vi "CRIO_State2String.vi"(8 "error in (no error)":errorcluster, 11 "Curr State":T1) -> (0 "error out":errorcluster, 3 "State Str":string)   [LabVIEW 2017]
uses:
  CRIO_StateEnum.ctl
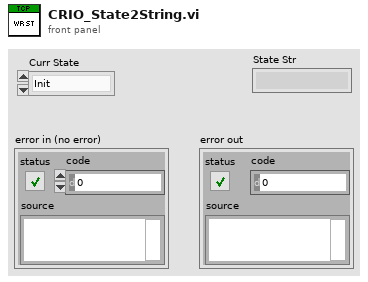
[diagram p1: front panel]
types:
  T1 = typedef "CRIO_StateEnum.ctl" = enum16{"Init", "Listen", "Wait", "Setup", "Ready to Launch", "Start Flight", "Accelerating", "Coasting", "Braking", "End Flight", "Loading", "Stop"}
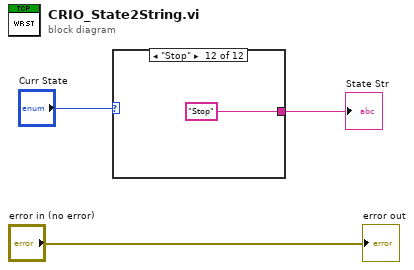
[diagram p0: block diagram]
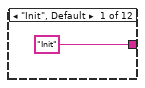
[diagram p2: hidden frame]
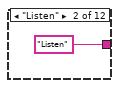
[diagram p3: hidden frame]
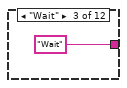
[diagram p4: hidden frame]
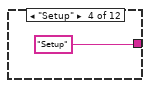
[diagram p5: hidden frame]
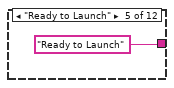
[diagram p6: hidden frame]
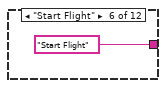
[diagram p7: hidden frame]
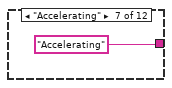
[diagram p8: hidden frame]
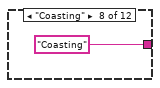
[diagram p9: hidden frame]
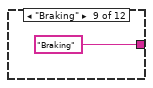
[diagram p10: hidden frame]
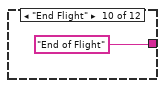
[diagram p11: hidden frame]
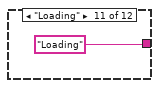
[diagram p12: hidden frame]
diagram:
  n1 = case shown="\"Stop\"" "Curr State" {
    tunnel: ["Init" ("y") "Listen" ("y") "Wait" ("y") "Setup" ("y") "Ready to Launch" ("y") "Start Flight" ("y") "Accelerating" ("y") "Coasting" ("y") "Braking" ("y") "End of Flight" ("y") "Loading" ("y") "Stop" ("y")] -> w1
    frame "Init", Default {
    }
    frame "Listen" {
    }
    frame "Wait" {
    }
    frame "Setup" {
    }
    frame "Ready to Launch" {
    }
    frame "Start Flight" {
    }
    frame "Accelerating" {
    }
    frame "Coasting" {
    }
    frame "Braking" {
    }
    frame "End Flight" {
    }
    frame "Loading" {
    }
    frame "Stop" {
    }
  }
  "State Str" <- w1
  "error out" <- "error in (no error)"
